vi "WFAppend.vi"(0 "Waveform In":waveform(dbl)={"t0"=timestamp(0 s since 1904-01-01), "dt"=0.0, "Y"=[]}, 1 "Waveform In 2":waveform(dbl)={"t0"=timestamp(0 s since 1904-01-01), "dt"=0.0, "Y"=[]}, 2 "Waveform In 3":waveform(dbl)={"t0"=timestamp(0 s since 1904-01-01), "dt"=0.0, "Y"=[]}, 3 "Waveform In 4":waveform(dbl)={"t0"=timestamp(0 s since 1904-01-01), "dt"=0.0, "Y"=[]}, 4 "Waveform In 5":waveform(dbl)={"t0"=timestamp(0 s since 1904-01-01), "dt"=0.0, "Y"=[]}, 5 "error in (no error)":errorcluster) -> (14 "Waveform Out":waveform(dbl), 19 "error out":errorcluster)   [LabVIEW 2013]
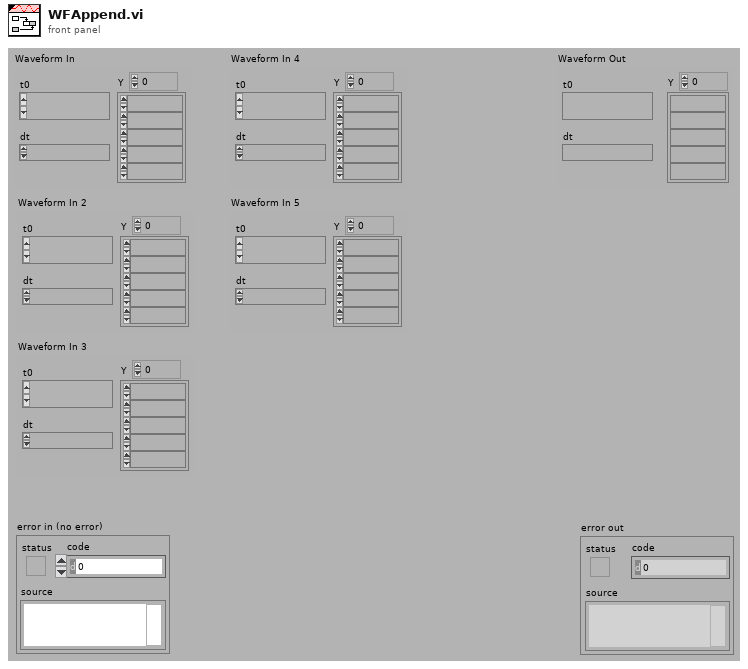
[diagram p1: front panel]
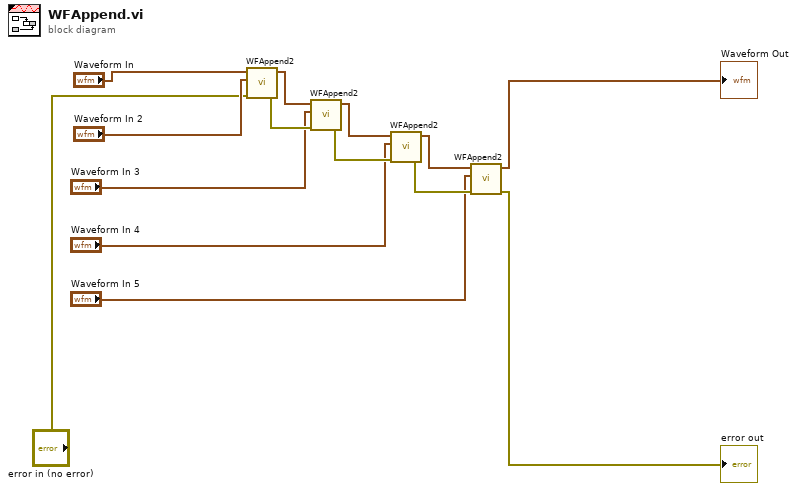
[diagram p0: block diagram]
diagram:
  n1 = call "WFAppend2.vi"("error in (no error)"="error in (no error)", "Waveform In 2"="Waveform In 2", "Waveform In"="Waveform In") -> ("error out"=w13:errorcluster, "Waveform Out"=w14:waveform(dbl))  [unwired: 3 in]
  n2 = call "WFAppend2.vi"("error in (no error)"=w13, "Waveform In 2"="Waveform In 3", "Waveform In"=w14) -> ("error out"=w11:errorcluster, "Waveform Out"=w12:waveform(dbl))  [unwired: 3 in]
  n3 = call "WFAppend2.vi"("error in (no error)"=w11, "Waveform In 2"="Waveform In 4", "Waveform In"=w12) -> ("error out"=w9:errorcluster, "Waveform Out"=w10:waveform(dbl))  [unwired: 3 in]
  n4 = call "WFAppend2.vi"("error in (no error)"=w9, "Waveform In 2"="Waveform In 5", "Waveform In"=w10) -> ("error out"=→"error out":errorcluster, "Waveform Out"=→"Waveform Out":waveform(dbl))  [unwired: 3 in]
